vi "UDP - Data ADC (SubVI).vi"(8 "error in (no error)":errorcluster, 11 "Data":string="\u0002|8ÿÿÿ\u0000\u0000\u0000\u0000\u0000\u0002\u0001\u0001\u0001\u0001\u0000ÈB¸\u0000\u0000\u0000\u0000\u0000zD\u0000\u0000 \u0000ÿÿÿ\u0000\u0000\u0000\u0000\u0000\u0000\u0000ð?\u0000\u0000\u0000\u0000\u0000\u0000ð?\u0000\u0000\u0000\u0000\u0000\u0000ð?\u0000\u0000\u0000\u0000\u0000\u0000ð?\u0000\u0000\u0000\u0000\u0000\u0000ð?\u0000\u0000\u0000\u0000\u0000\u0000ð?\u0000\u0000\u0000\u0000\u0000\u0000ð?\u0000\u0000\u0000\u0000\u0000\u0000ð?\u0000\u0000\u0000 …ëó?\u0000\u0000\u0000 …ëó?\u0000\u0000\u0010\u0000\u0000\u0000\u0000\u0000z") -> (0 "error out":errorcluster, 3 "Data ADC":T1, 4 "Success":bool)   [LabVIEW 2019]
panel:
  in  "Data 2":string="\u0002|8ÿÿÿ\u0000\u0000\u0000\u0000\u0000\u0002\u0001\u0001\u0001\u0001\u0000ÈB¸\u0000\u0000\u0000\u0000\u0000zD\u0000\u0000 \u0000ÿÿÿ\u0000\u0000\u0000\u0000\u0000\u0000\u0000ð?\u0000\u0000\u0000\u0000\u0000\u0000ð?\u0000\u0000\u0000\u0000\u0000\u0000ð?\u0000\u0000\u0000\u0000\u0000\u0000ð?\u0000\u0000\u0000\u0000\u0000\u0000ð?\u0000\u0000\u0000\u0000\u0000\u0000ð?\u0000\u0000\u0000\u0000\u0000\u0000ð?\u0000\u0000\u0000\u0000\u0000\u0000ð?\u0000\u0000\u0000 …ëó?\u0000\u0000\u0000 …ëó?\u0000\u0000\u0010\u0000\u0000\u0000\u0000\u0000z"
  out "subarray 2":u8[](array[numeric]) format="%.0x"
  out "subarray":u8[](array[numeric]) format="%.0x"
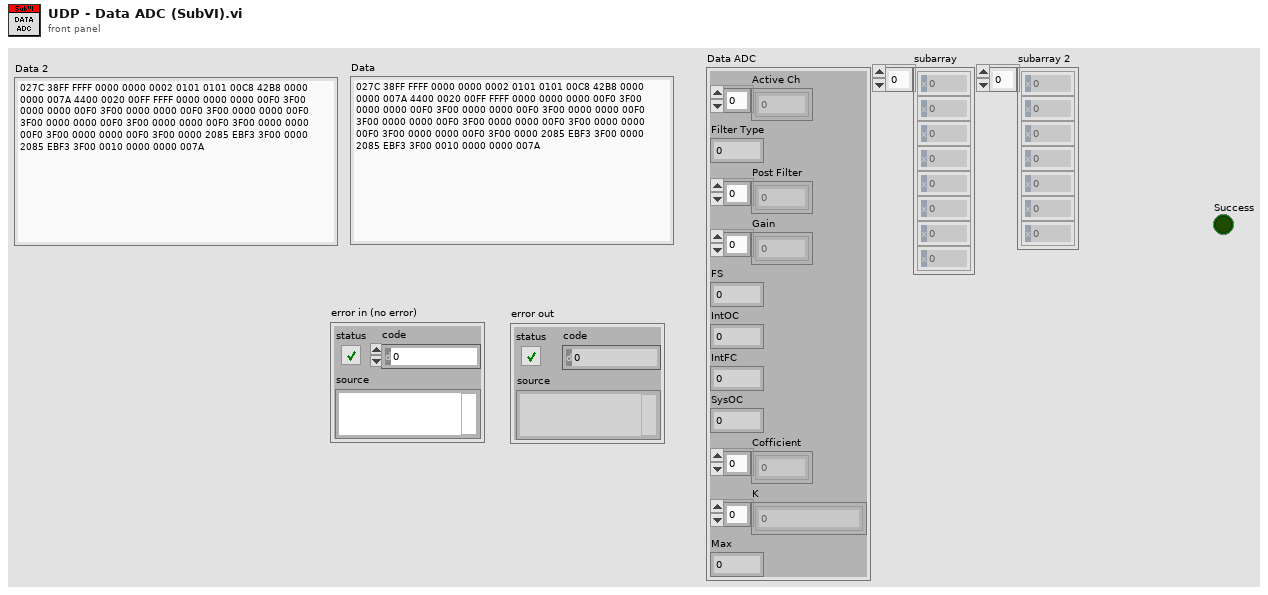
[diagram p1: front panel]
types:
  T1 = cluster{"Active Ch":u8[], "Filter Type":u8, "Post Filter":u8[], "Gain":u8[], "FS":u16, "IntOC":u8, "IntFC":u8, "SysOC":u8, "Cofficient":dbl[], "K":dbl[], "Max":i32}
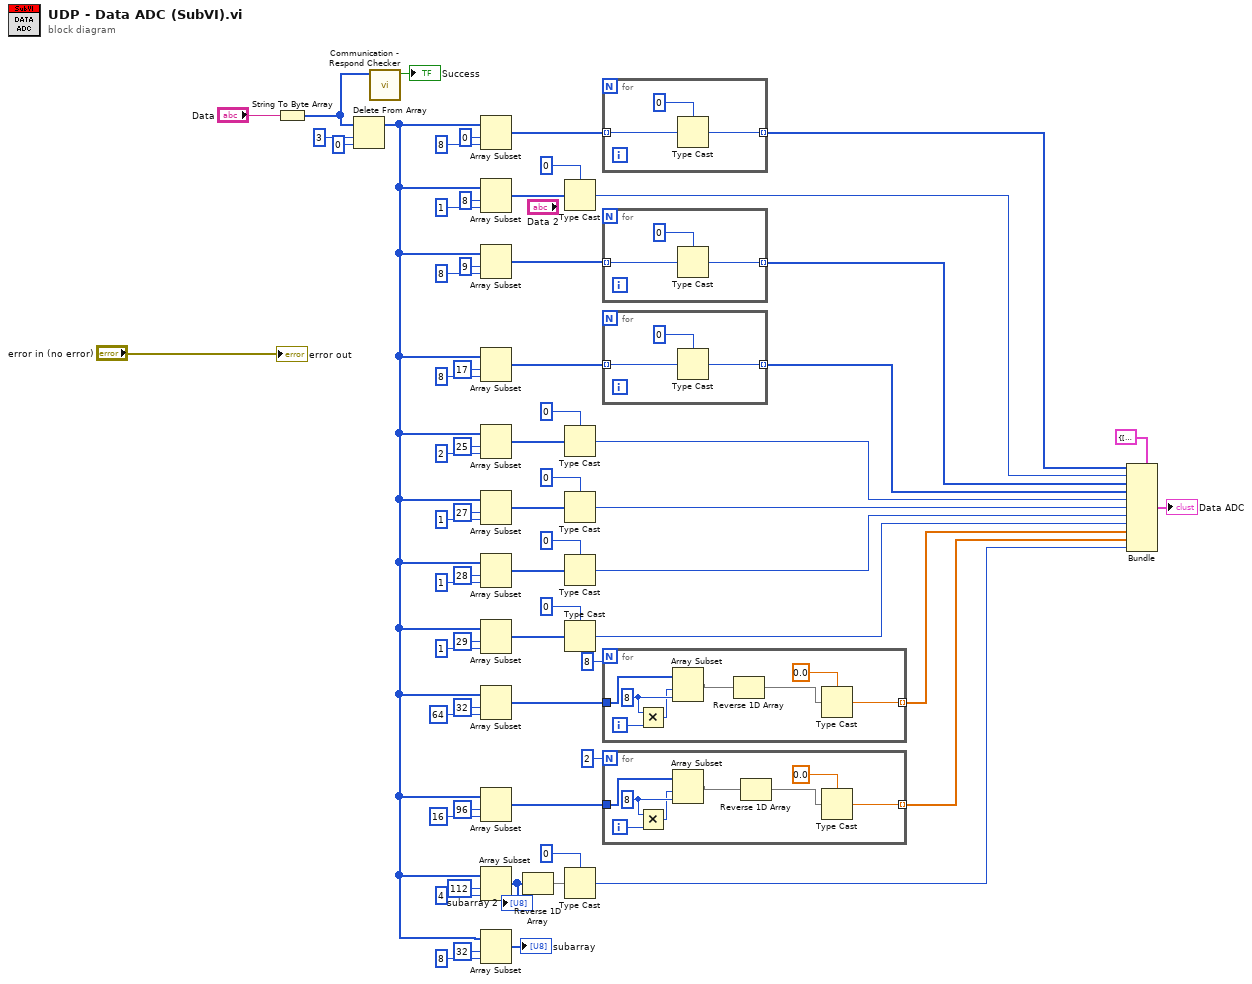
[diagram p0: block diagram]
diagram:
  n1 = String To Byte Array(string="Data") -> (unsigned byte array=w32:u8[])
  n2 = Delete From Array(array=w32, length=3, index=0) -> (array with subset deleted=w3:u8[])  [unwired: 1 out]
  n3 = call "Communication - Respond Checker.vi"("Read Data"=w32) -> ("Success"=→"Success":bool)  [unwired: 10 in]
  n4 = Array Subset(array=w3, index=0, length=8) -> (w31:u8[])
  n5 = Array Subset(array=w3, index=8, length=1) -> (w30:u8[])
  n6 = Array Subset(array=w3, index=9, length=8) -> (w29:u8[])
  n7 = Array Subset(array=w3, index=17, length=8) -> (w28:u8[])
  n8 = Array Subset(array=w3, index=25, length=2) -> (w27:u8[])
  n9 = Array Subset(array=w3, index=27, length=1) -> (w24:u8[])
  n10 = Array Subset(array=w3, index=28, length=1) -> (w25:u8[])
  n11 = Array Subset(array=w3, index=29, length=1) -> (w26:u8[])
  n12 = Array Subset(array=w3, index=32, length=64) -> (w22:u8[])
  n13 = Array Subset(array=w3, index=96, length=16) -> (w20:u8[])
  n14 = Array Subset(array=w3, index=112, length=4) -> (w6:u8[])
  "subarray 2" <- w6
  n15 = Array Subset(array=w3, index=32, length=8) -> (→"subarray":u8[])
  n16 = Reverse 1D Array(array=w6) -> (reversed array=w1:u8[])
  n17 = Type Cast(type=u8 0, x=w30) -> (*(type *) &x=w17:u8)
  n18 = Type Cast(type=u16 0, x=w27) -> (*(type *) &x=w14:u16)
  n19 = Type Cast(type=u8 0, x=w24) -> (*(type *) &x=w13:u8)
  n20 = Type Cast(type=u8 0, x=w25) -> (*(type *) &x=w12:u8)
  n21 = Type Cast(type=u8 0, x=w26) -> (*(type *) &x=w11:u8)
  n22 = Type Cast(type=0, x=w1) -> (*(type *) &x=w8:i32)
  n23 = for {
    tunnel: [w67] -> w18 mode=indexing
    tunnel: w31 -> [w66] mode=indexing
    n24 = Type Cast(type=u8 0, x=w66) -> (*(type *) &x=w67:u8)
  }
  n25 = for {
    tunnel: [w70] -> w16 mode=indexing
    tunnel: w29 -> [w69] mode=indexing
    n26 = Type Cast(type=u8 0, x=w69) -> (*(type *) &x=w70:u8)
  }
  n27 = for {
    tunnel: [w73] -> w15 mode=indexing
    tunnel: w28 -> [w72] mode=indexing
    n28 = Type Cast(type=u8 0, x=w72) -> (*(type *) &x=w73:u8)
  }
  n29 = for {
    N: 8 -> [_]
    tunnel: [w81] -> w10 mode=indexing
    tunnel: w22 -> [w80]
    i -> [w79]
    w78 = 8 ("length")
    n30 = Multiply(x=w78, y=w79) -> (x*y=w77:i32)
    n31 = Array Subset(array=w80, index=w77, length=w78) -> (w76:u8[])
    n32 = Reverse 1D Array(array=w76) -> (reversed array=w75:u8[])
    n33 = Type Cast(type=0.0, x=w75) -> (*(type *) &x=w81:dbl)
  }
  n34 = for {
    N: 2 -> [_]
    tunnel: [w89] -> w9 mode=indexing
    tunnel: w20 -> [w88]
    i -> [w87]
    w86 = 8 ("length")
    n35 = Multiply(x=w86, y=w87) -> (x*y=w85:i32)
    n36 = Array Subset(array=w88, index=w85, length=w86) -> (w84:u8[])
    n37 = Reverse 1D Array(array=w84) -> (reversed array=w83:u8[])
    n38 = Type Cast(type=0.0, x=w83) -> (*(type *) &x=w89:dbl)
  }
  n39 = Bundle(cluster=T1 {"Active Ch"=[255, 255, 255, 0, 0, 0, 0, 0], "Filter Type"=2, "Post Filter"=[1, 1, 1, 1, 0, 200, 66, 184], "Gain"=[0, 0, 0, 0, 0, 122, 68, 0], "FS"=32, "IntOC"=0, "IntFC"=255, "SysOC"=255, "Cofficient"=[1.0, 1.0, 1.0, 1.0, 1.0, 1.0, 1.0, 1.0], "K"=[1.2450000047683716, 1.2450000047683716], "Max"=1048576}, "Active Ch"=w18, "Filter Type"=w17, "Post Filter"=w16, "Gain"=w15, "FS"=w14, "IntOC"=w13, "IntFC"=w12, "SysOC"=w11, "Cofficient"=w10, "K"=w9, "Max"=w8) -> (→"Data ADC":T1)
  "error out" <- "error in (no error)"
